vi "CH_LM Test Status.vi"() -> ()   [LabVIEW 2012, in "CH_LM.lvlib"]
doc: "This VI reads the current software revisions and meter information once.\nThen it reads periodically the probe information and system status."
uses:
  CH_LM.lvlib
  CH_LM/CH_LM ProbeType.ctl
  CH_LM/CH_LM ProbeQualifier.ctl
  CH_LM/CH_LM Meter Type.ctl
  CH_LM/CH_LM Date Format.ctl
  CH_LM/CH_LM System StatusCluster.ctl
  CH_LM/CH_LM BaudRates.ctl
  CH_LM/CH_LM Parity.ctl
  CH_LM/CH_LM SerialConfiguration.ctl
panel:
  in  "Serial Configuration\n(19200,N,8,1)":T1={"Baud Rate"=19200, "Parity"=0, "Data Bits"=8, "Stop Bits"=1} {"Parity" items=["None", "Odd", "Even"]; "Baud Rate" items=["9600"=9600, "19200"=19200, "38400"=38400, "57600"=57600, "115200"=115200]}
  out "Probe Diameter":dbl[unit] format="%#.2g"
  out "Probe Qualifier":T4
  out "stopped":bool
  out "last update":timestamp
  out "loop":i32
  out "Status Description":string
  out "Probe Serial Number":string
  out "Head Temperature":dbl[unit]=273.15
  out "P Calibration Date":timestamp format="%<%x>T"
  out "Responsitivity":dbl format="%#.1g"
  out "Probe Type":T5
  out "Model":string
  in  "Reset":bool
  out "error out":errorcluster
  in  "stop":bool
  out "Meter Serial Number":string
  out "M Calibration Date":string
  out "Time Stamp":timestamp format="%<%X\n%x>T"
  out "Date Format":T6
  out "Meter Type":T7
  out "Instrument Firmware Date":string
  out "Instrument Firmware Revision":string
  out "Instrument Driver Revision":string
  out "Vendor":string
  out "Module":string
  out "Status":T8
  out "timed out?":bool
  in  "Address":i32=1
  in  "Serial Number":string
  in  "Reset? (F: No)":bool
  in  "ID Query? (T: Yes)":bool
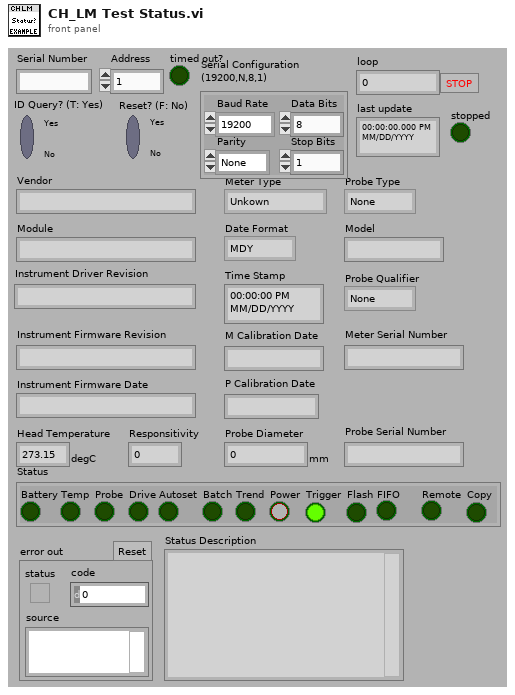
[diagram p1: front panel]
types:
  T1 = typedef "CH_LM.lvlib/CH_LM SerialConfiguration.ctl" = cluster{"Baud Rate":T2, "Parity":T3, "Data Bits":u16, "Stop Bits":u16}
  T2 = typedef "CH_LM.lvlib/CH_LM BaudRates.ctl" = u32
  T3 = typedef "CH_LM.lvlib/CH_LM Parity.ctl" = u16
  T4 = typedef "CH_LM.lvlib/CH_LM ProbeQualifier.ctl" = enum16{"None", "Single", "Quad", "No Spec"}
  T5 = typedef "CH_LM.lvlib/CH_LM ProbeType.ctl" = enum16{"None", "Thermopile", "Pyroelectric", "Optical"}
  T6 = typedef "CH_LM.lvlib/CH_LM Date Format.ctl" = enum16{"MDY", "DMY"}
  T7 = typedef "CH_LM.lvlib/CH_LM Meter Type.ctl" = enum16{"Unkown", "TOP", "TO"}
  T8 = typedef "CH_LM.lvlib/CH_LM System StatusCluster.ctl" = cluster{"Battery":bool, "Temp":bool, "Probe":bool, "Drive":bool, "Autoset":bool, "Batch":bool, "Trend":bool, "Power":bool, "Trigger":bool, "Flash":bool, "FIFO":bool, "Remote":bool, "Copy":bool}
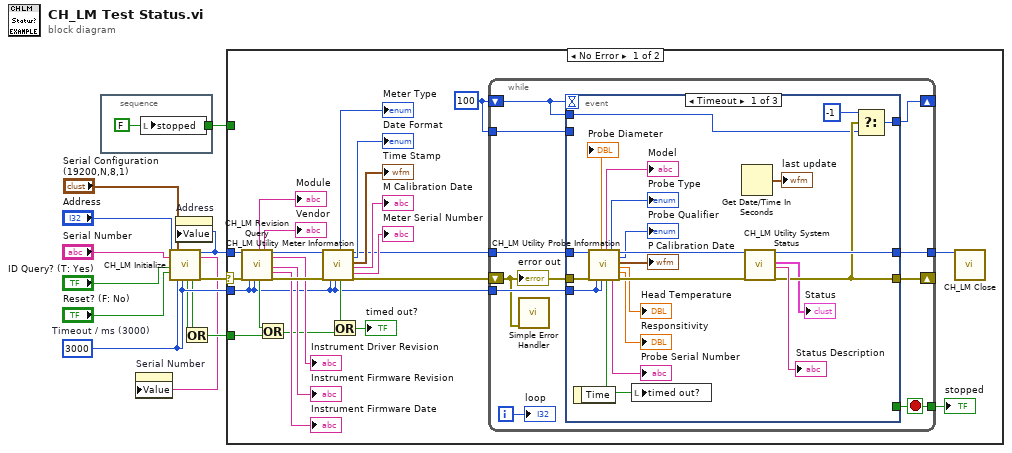
[diagram p0: block diagram]
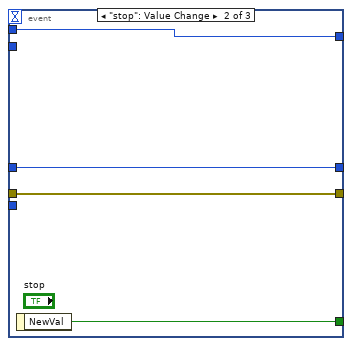
[diagram p2: hidden frame]
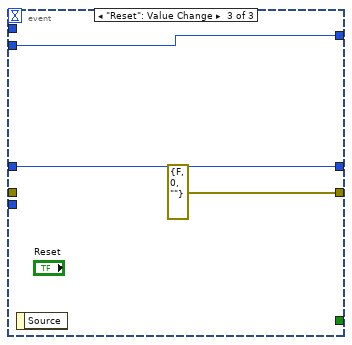
[diagram p3: hidden frame]
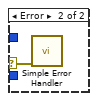
[diagram p4: hidden frame]
diagram:
  w10 = 3000  # Timeout / ms (3000)
  n1 = stacked-sequence {
    tunnel: [w14] -> w6
    frame #0 {
      w14 = FALSE ("stopped")
      n2 = local write "stopped"(w14) -> ()
    }
  }
  n3 = call "CH_LM Initialize.vi"("Address"="Address", "Serial Number"="Serial Number", "ID Query (True)"="ID Query? (T: Yes)", "Reset (False)"="Reset? (F: No)", "Serial Configuration\n(19200,N,8,1)"="Serial Configuration\n(19200,N,8,1)", "Timeout / ms (3000)"=w10, "Lock Timeout / ms (1000)"=w10) -> ("Lock timed out"=w9:bool, "timed out?"=w8:bool, "Meter Index"=w3:i32, "Serial Number"=w2:string, "error out"=w11:errorcluster)  [unwired: 1 in, 7 out]
  n4 = property on="Serial Number" class="Str"("Value"=w2) -> ()  [unwired: 2 in, 2 out]
  n5 = property on="Address" class="DigNum (strict)"("Value"=w3) -> ()  [unwired: 2 in, 2 out]
  n6 = Or(x=w8, y=w9) -> (x .or. y?=w7:bool)
  n7 = case shown="No Error" w11 {
    selector: w11 -> [w38 w79]
    tunnel: w3 -> [w39 _]
    tunnel: w10 -> [w17 _]
    tunnel: w7 -> [w30 _]
    tunnel: w6 -> [_ _]
    frame No Error {
      w15 = 100
      n8 = call "CH_LM Revision Query.vi"("Meter Index"=w39, "error in (no error)"=w38, "Timeout / ms (3000)"=w17, "Lock Timeout / ms (1000)"=w17) -> ("Module"=→"Module":string, "Lock timed out"=w29:bool, "Vendor"=→"Vendor":string, "Meter Index"=w37:i32, "Instrument Driver Revision"=→"Instrument Driver Revision":string, "Instrument Firmware Revision"=→"Instrument Firmware Revision":string, "Instrument Firmware Date"=→"Instrument Firmware Date":string, "error out"=w36:errorcluster)  [unwired: 8 out]
      n9 = Or(x=w29, y=w30) -> (x .or. y?=w22:bool)
      n10 = call "CH_LM Utility Meter Information.vi"("Meter Index"=w37, "error in (no error)"=w36, "Timeout / ms (3000)"=w17, "Lock Timeout / ms (1000)"=w17) -> ("Lock timed out"=w23:bool, "Meter Type"=→"Meter Type":T7, "Serial Number"=→"Meter Serial Number":string, "Meter Index"=w20:i32, "Date Format"=→"Date Format":T6, "Time Stamp"=→"Time Stamp":timestamp, "Calibration Date"=→"M Calibration Date":string, "error out"=w19:errorcluster)  [unwired: 3 in, 5 out]
      n11 = Or(x=w23, y=w22) -> (x .or. y?=→"timed out?":bool)
      n12 = while {
        tunnel: w20 -> [w49]
        tunnel: [w48] -> w18
        shift-right: [w47] -> _
        shift-left: w19 -> [w40]
        tunnel: w17 -> [w46]
        tunnel: [w44] -> w16
        shift-right: [w43] -> _
        shift-left: w15 -> [w42]
        tunnel: w15 -> [w41]
        i -> [w45]
        stop <- w44 stop-if-true
        n13 = call <vilib>:"Simple Error Handler.vi"("error in (no error)"=w40) -> ()  [unwired: 1 in, 8 out]
        n14 = event shown="[0] Timeout" {
          selector: _ -> [_ _ _]
          dyn-events: _ -> [_ _ _]
          timeout: w42 -> [_ _ _]
          tunnel: [_ w75 _] -> w44
          tunnel: w49 -> [w70 w74 w77]
          tunnel: w40 -> [w69 w73 _]
          tunnel: [w59 w74 w77] -> w48
          tunnel: [w57 w73 errorcluster {"status"=FALSE, "code"=0, "source"=""} ("error out")] -> w47
          tunnel: w46 -> [w62 _ _]
          tunnel: [w56 w72 w76] -> w43
          tunnel: w42 -> [w55 w72 _]
          tunnel: w41 -> [_ _ w76]
          event Timeout {
            n15 = event-data() -> ()  [unwired: 2 out]
            n16 = call "CH_LM Utility Probe Information.vi"("Meter Index"=w70, "error in (no error)"=w69, "Timeout / ms (3000)"=w62, "Lock Timeout / ms (1000)"=w62) -> ("Probe Diameter"=→"Probe Diameter":dbl[unit], "Model"=→"Model":string, "Lock timed out"=w61:bool, "Probe Type"=→"Probe Type":T5, "Serial Number"=→"Probe Serial Number":string, "Meter Index"=w71:i32, "Probe Qualifier"=→"Probe Qualifier":T4, "Calibration Date"=→"P Calibration Date":timestamp, "Head Temperature"=→"Head Temperature":dbl[unit], "Responsitivity"=→"Responsitivity":dbl, "error out"=w68:errorcluster)  [unwired: 5 out]
            n17 = local write "timed out?"(w61) -> ()
            n18 = Get Date/Time In Seconds() -> (seconds since 1Jan1904=→"last update":timestamp)
            n19 = call "CH_LM Utility System Status.vi"("Meter Index"=w71, "error in (no error)"=w68) -> ("Meter Index"=w59:i32, "Status"=→"Status":T8, "Status Description"=→"Status Description":string, "error out"=w57:errorcluster)  [unwired: 14 out]
            n20 = Select(t=-1, s=w57, f=w55) -> (s? t:f=w56:i32)
          }
          event "stop": Value Change {
            n21 = event-data() -> ("NewVal"=w75:bool)  [unwired: 1 out]
          }
          event "Reset": Value Change {
            n22 = event-data() -> ()  [unwired: 2 out]
          }
        }
        "error out" <- w40
        "loop" <- w45
      }
      "stopped" <- w16
      n23 = call "CH_LM Close.vi"("Meter Index"=w18) -> ()  [unwired: 1 in, 18 out]
    }
    frame Error {
      n24 = call <vilib>:"Simple Error Handler.vi"("error in (no error)"=w79) -> ()  [unwired: 1 in, 8 out]
    }
  }
